vi "Read Gas Ref.vi"(8 "error in (no error)":errorcluster, 11 "DMA in":refnum<class "DMA.lvclass">) -> (0 "error out":errorcluster, 2 "Gas Ref":refnum<data-value>, 3 "DMA out":refnum<class "DMA.lvclass">)   [LabVIEW 2014, in "DMA.lvclass"]
uses:
  DMA.lvclass
  Atmospheric/Gas Properties/Gas Properties.lvclass
  DMA.lvclass/DMA.ctl
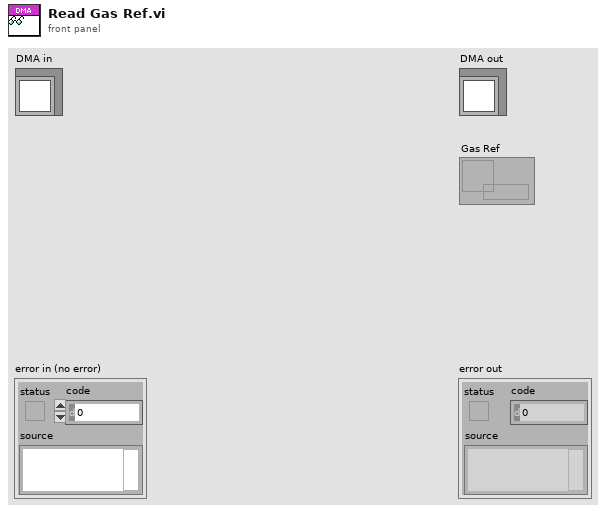
[diagram p1: front panel]
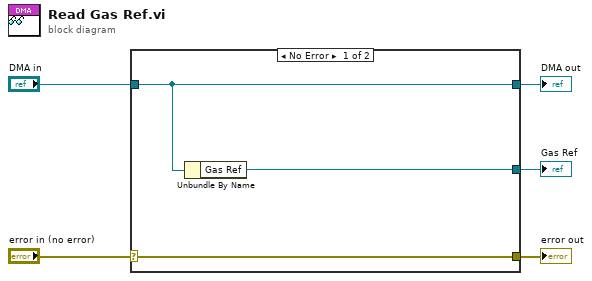
[diagram p0: block diagram]
diagram:
  n1 = case shown="No Error" "error in (no error)" {
    selector: "error in (no error)" -> [w8 w9]
    tunnel: [w8 w9] -> w4
    tunnel: [w7 w10] -> w2
    tunnel: "DMA in" -> [w7 w10]
    tunnel: [w6 _] -> w1
    frame No Error {
      n2 = Unbundle By Name(w7) -> ("Gas Ref"=w6:refnum<data-value>)
    }
    frame Error {
    }
  }
  "error out" <- w4
  "DMA out" <- w2
  "Gas Ref" <- w1
